vi "Main.vi"(11 "Module Admin":refnum<class "Delacor_lib_QMH_Module Admin.lvclass">) -> ()   [LabVIEW 2024, in "Coffee Prefers.lvlib"]
doc: "This template is based off of the Queued Message Handler design pattern and the Queued Message Handler project template that ships with LabVIEW.\n\nThe main difference is that the queue is private to this module and communication between modules is performed via Broadcast and Request events.\n\nRequest events are wrapped in public API methods and are handled in the Event Handling Loop (EHL) of this VI. Any module can register for Broadcast events sent by this module. The EHL generates messages based on user interface actions.\n\nThe Message Handling Loop (MHL) processes messages generated by the EHL, or by other messages. The messages are string values, so new messages can be added easily to the Message Cases case structure in the MHL. Each message cluster can also provide an optional value for Message Data, which is a variant that can be converted to whatever message-specific data is required.\n_____\nBased on DQMH Project Template 7.0.1.1316."
uses:
  Coffee Prefers.lvlib
  <vilib>/Delacor/Delacor QMH/Libraries/Module Admin_class/Delacor_lib_QMH_Module Admin.lvclass
  choose coffee--combobox.ctl
  Module Data--cluster.ctl
  <vilib>/Delacor/Delacor QMH/Libraries/Message Queue_class/Delacor_lib_QMH_Message Queue.lvclass/Delacor_lib_QMH_Message Queue.ctl
  Stop Argument--cluster.ctl
  <vilib>/Delacor/Delacor QMH/Libraries/Module Admin_class/Delacor_lib_QMH_Module Admin.lvclass/Delacor_lib_QMH_Module Admin.ctl
  user inputs--cluster.ctl
  Material broadcast -- cluster.ctl
  <vilib>/Utility/miscctls.llb/LVPointTypeDef.ctl
  <vilib>/Delacor/Delacor QMH/Libraries/Message Queue_class/Delacor_lib_QMH_Enqueue Message (Single).vi
  <vilib>/Delacor/Delacor QMH/Libraries/Module Admin_class/Delacor_lib_QMH_Get External Launch.vi
  <vilib>/Delacor/Delacor QMH/Libraries/Message Queue_class/Delacor_lib_QMH_Message Queue.lvclass
  Tank/Tank.lvlib
panel:
  in  "Milk intensity":dbl
  in  "Coffe intensity":dbl
  in  "Choose Coffe":T1
  out "error out":errorcluster
  out "Status":string
  in  "Simulate MHL Error":bool
  in  "Simulate EHL Error":bool
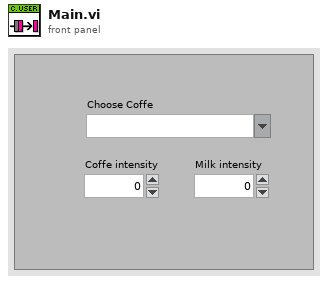
[diagram p1: front panel]
types:
  T1 = typedef "Coffee Prefers.lvlib/choose coffee--combobox.ctl" = string
  T2 = typedef "Coffee Prefers.lvlib/Request Events--cluster.ctl" = cluster{"Stop Module":refnum<user-event>, "Show Panel":refnum<user-event>, "Hide Panel":refnum<user-event>, "Get Module Execution Status":refnum<user-event>, "Show Diagram":refnum<user-event>}
  T3 = typedef "Tank.lvlib/Broadcast Events--cluster.ctl" = cluster{"Module Did Init":refnum<user-event>, "Status Updated":refnum<user-event>, "Error Reported":refnum<user-event>, "Module Did Stop":refnum<user-event>, "Update Module Execution Status":refnum<user-event>, "Tank Situation":refnum<user-event>}
  T4 = typedef "Coffee Prefers.lvlib/Module Data--cluster.ctl" = cluster{"Status":string, "Coffee":i16, "Milk":i16, "Water":i16, "milk intensity":dbl, "coffee instensity":dbl, "choose coffe":string}
  T5 = enum32{"invalid lock state", "Not Locked", "Locked (No Password)", "Password-protected"}
  T6 = typedef "Coffee Prefers.lvlib/Stop Argument--cluster.ctl" = cluster{"Origin":string, "Exit via Stop Module Req?":bool, "Wait for Module to stop?":bool}
  T7 = typedef "Coffee Prefers.lvlib/user inputs--cluster.ctl" = cluster{"choose coffe":string, "coffee instensity":dbl, "milk intensity":dbl}
  T8 = typedef "Material broadcast -- cluster.ctl" = cluster{"Coffee":i32, "Milk":i32, "Water":i32}
  T9 = typedef "LVPointTypeDef.ctl" = cluster{"Horizontal":i16, "Vertical":i16}
  T10 = enum32{"Invalid", "Standard", "Closed", "Hidden", "Minimized", "Maximized"}
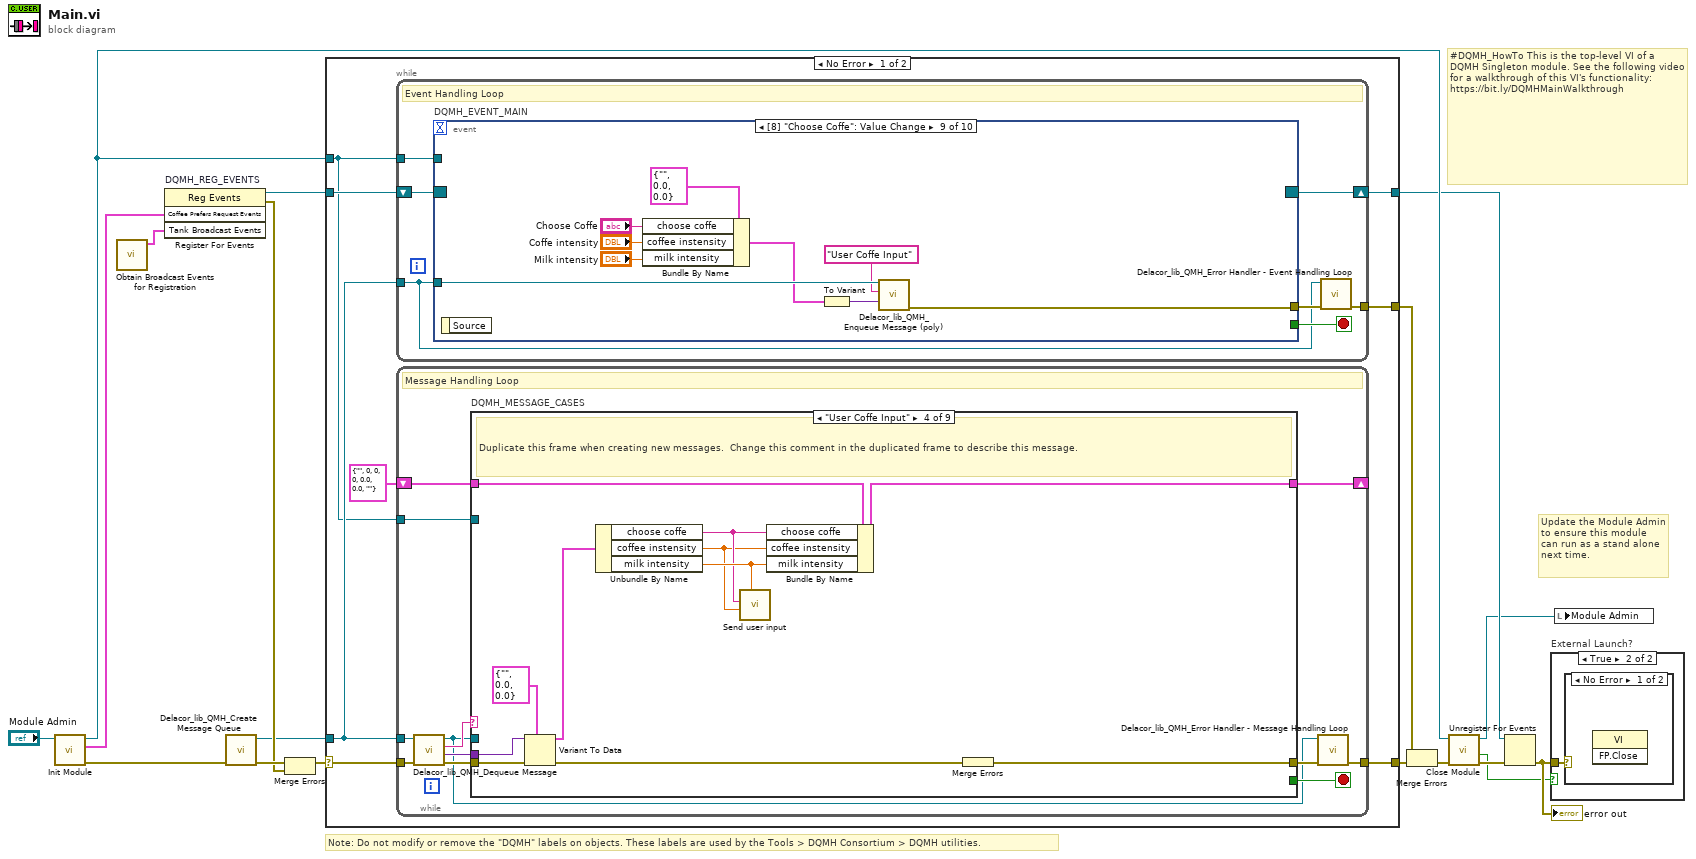
[diagram p0: block diagram]
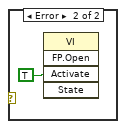
[diagram p3: hidden frame]
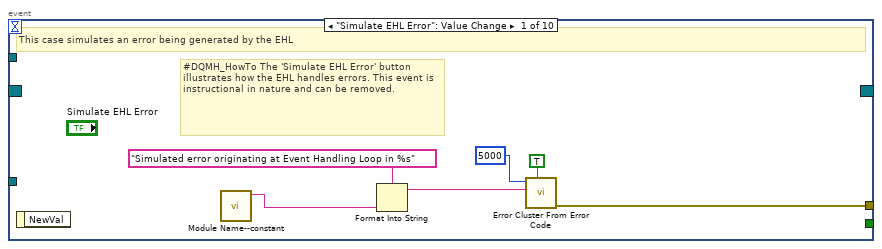
[diagram p4: hidden frame]
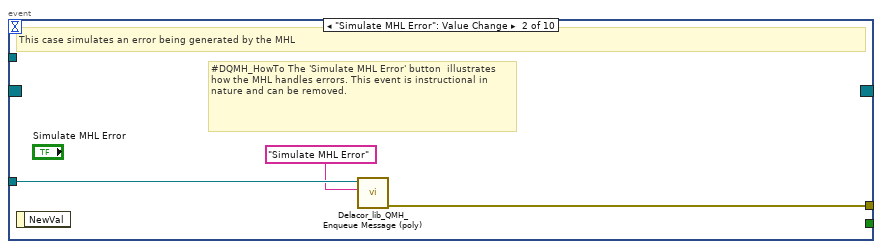
[diagram p5: hidden frame]
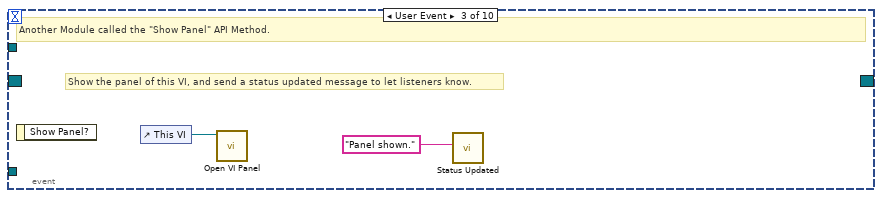
[diagram p6: hidden frame]
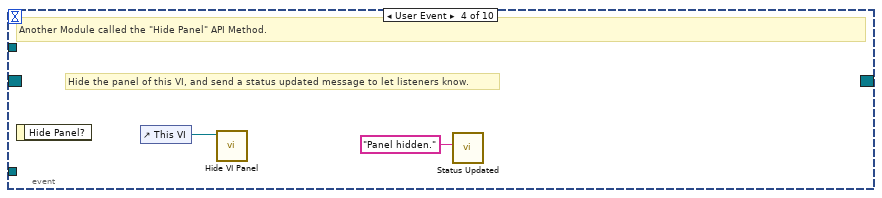
[diagram p7: hidden frame]
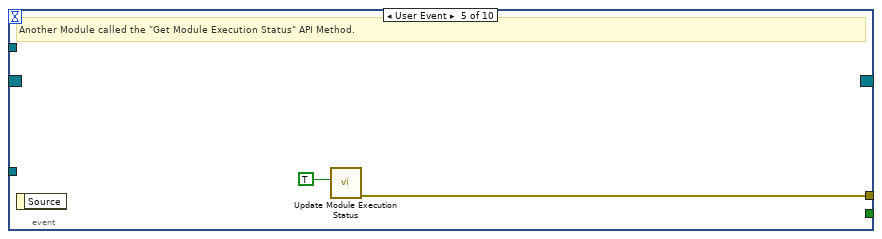
[diagram p8: hidden frame]
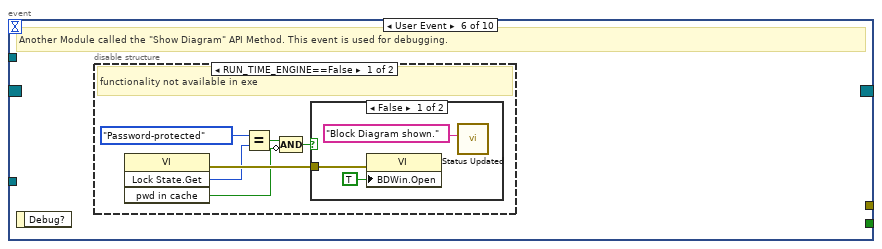
[diagram p9: hidden frame]
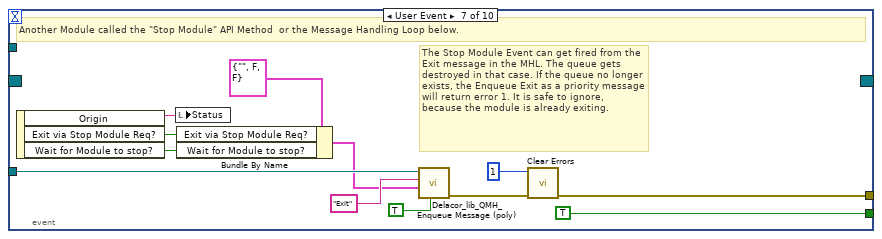
[diagram p12: hidden frame]
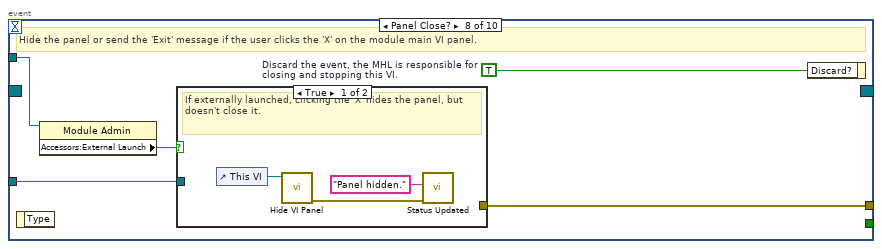
[diagram p13: hidden frame]
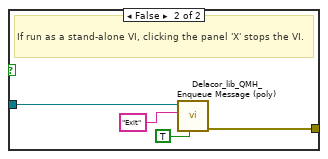
[diagram p14: hidden frame]
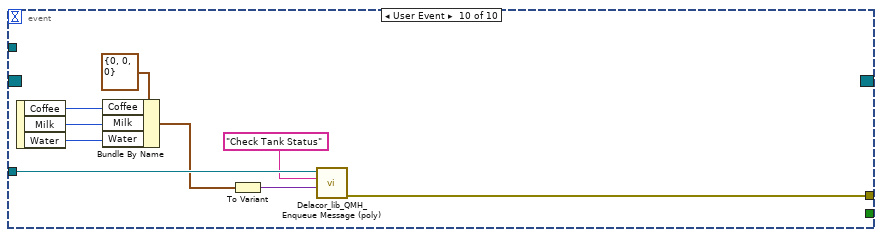
[diagram p15: hidden frame]
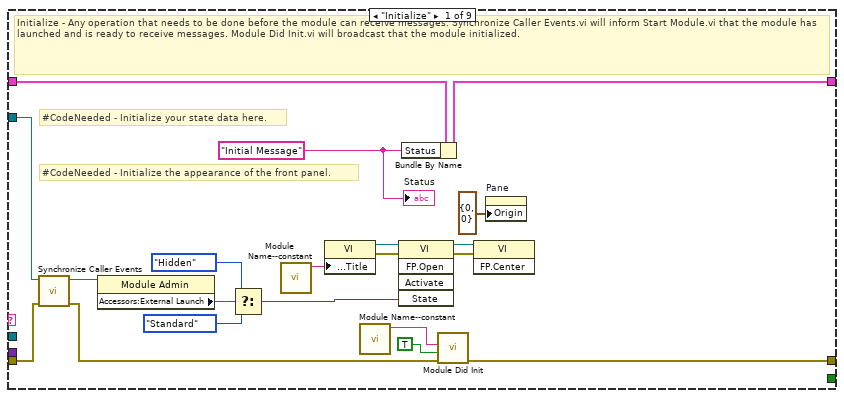
[diagram p16: hidden frame]
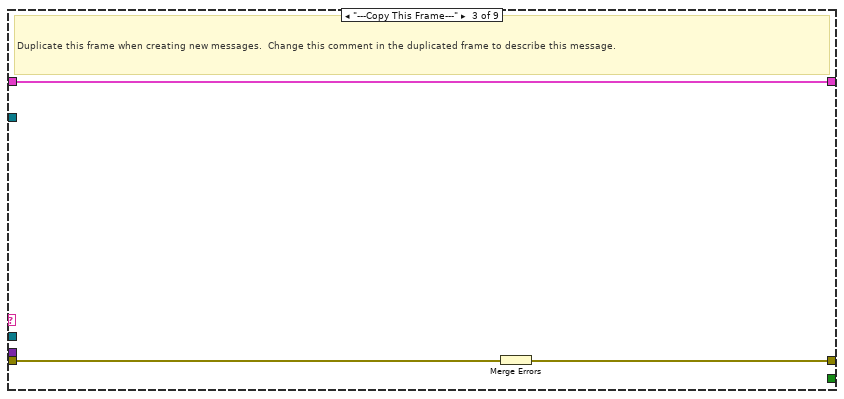
[diagram p18: hidden frame]
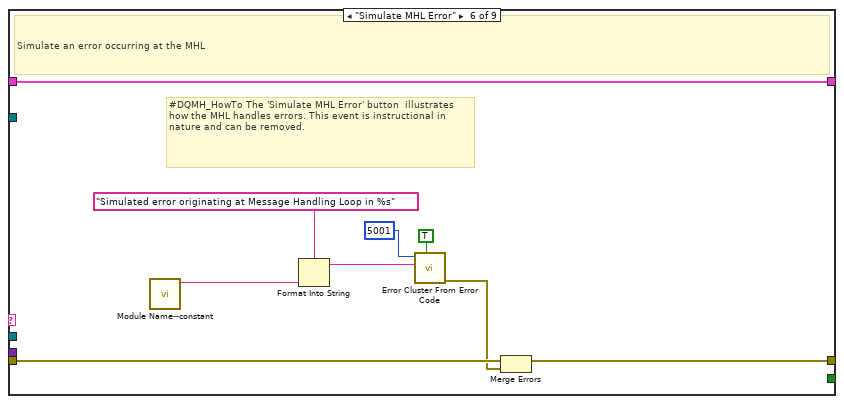
[diagram p20: hidden frame]
diagram:
  # "#DQMH_HowTo This is the top-level VI of a DQMH Singleton module. See the following video for a walkthrough of this VI's functionality: https://bit.ly/DQMHMainWalkthrough"
  # "Note: Do not modify or remove the \"DQMH\" labels on objects. These labels are used by the Tools > DQMH Consortium > DQMH utilities."
  # "Update the Module Admin to ensure this module can run as a stand alone next time."
  n1 = call "Init Module.vi"("Singleton Module Admin in"="Module Admin") -> ("error out"=w17:errorcluster, "Coffee Prefers Request Events"=w6:T2, "Singleton Module Admin out"=w9:refnum<class "Delacor_lib_QMH_Module Admin.lvclass">)  [unwired: 8 in]
  n2 = call "Obtain Broadcast Events for Registration.vi"() -> ("Tank Broadcast Events"=w1:T3)  [unwired: 9 in, 2 out]
  n3 = register-events "DQMH_REG_EVENTS"(w6, w1) -> (reference out=w7:refnum<event-registration>, error out=w10:errorcluster)  [unwired: 2 in]
  n4 = call <vilib>:"Delacor_lib_QMH_Create Message Queue.vi"("error in"=w17) -> ("error out"=w12:errorcluster, "Message Queue"=w5:refnum<class "Delacor_lib_QMH_Message Queue.lvclass">)  [unwired: 9 in]
  n5 = Merge Errors(w12, w10) -> (w11:errorcluster)
  n6 = case shown="No Error" w11 {
    selector: w11 -> [w24 w208]
    tunnel: [w26 w207] -> w18
    tunnel: [w23 w206] -> w8
    tunnel: w7 -> [w21 w206]
    tunnel: w5 -> [w20 w201]
    tunnel: [w25 _] -> w15
    tunnel: w9 -> [w19 w202]
    frame No Error {
      n7 = while {
        tunnel: w20 -> [w27]
        shift-right: [w30] -> w23
        shift-left: w21 -> [w31]
        tunnel: [w32] -> w25
        tunnel: w19 -> [w28]
        stop <- w29 stop-if-true
        # "Event Handling Loop"
        n8 = event "DQMH_EVENT_MAIN" shown="[8] \"Choose Coffe\": Value Change" {
          selector: w31 -> [_ _ _ _ _ _ _ _ _ _]
          dyn-events: [_ _ _ _ _ _ _ _ _ _] -> w30
          timeout: _ -> [_ _ _ _ _ _ _ _ _ _]
          tunnel: [_ _ _ _ _ _ TRUE ("Discard?") _ _ _] -> w29
          tunnel: w27 -> [_ w41 _ _ _ _ w65 w72 w90 w99]
          tunnel: [w39 w42 _ _ w48 _ w68 w74 w89 w98] -> w33
          tunnel: w28 -> [_ _ _ _ _ _ _ w71 _ _]
          event "Simulate EHL Error": Value Change {
            # "#DQMH_HowTo The 'Simulate EHL Error' button  illustrates how the EHL handles errors. This event is instructional in nature and can be removed."
            # "This case simulates an error being generated by the EHL"
            n9 = event-data() -> ()  [unwired: 1 in, 1 out]
            n10 = call "Module Name--constant.vi"() -> ("Module Name"=w36:string)  [unwired: 11 in]
            n11 = Format Into String(format string="Simulated error originating at Event Handling Loop in %s", w36) -> (resulting string=w37:string)  [unwired: 2 in, 1 out]
            n12 = call <vilib>:"Error Cluster From Error Code.vi"("show call chain? (False)"=TRUE, "error message (\"\")"=w37, "error code (0)"=5000) -> ("error out"=w39:errorcluster)  [unwired: 6 in]
          }
          event "Simulate MHL Error": Value Change {
            # "#DQMH_HowTo The 'Simulate MHL Error' button  illustrates how the MHL handles errors. This event is instructional in nature and can be removed."
            # "This case simulates an error being generated by the MHL"
            n13 = event-data() -> ()  [unwired: 1 in, 1 out]
            n14 = call-poly <vilib>:"Delacor_lib_QMH_Enqueue Message (poly).vi"("Message"="Simulate MHL Error", "Message Queue in"=w41) -> ("error out"=w42:errorcluster)  [unwired: 8 in, 1 out]
          }
          event User Event {
            # "Show the panel of this VI, and send a status updated message to let listeners know."
            # "Another Module called the \"Show Panel\" API Method."
            n15 = event-data() -> ()  [unwired: 1 in, 1 out]
            n16 = control-ref of="This VI"() -> (w44:refnum<vi>)
            n17 = call "Open VI Panel.vi"("VI"=w44) -> ()  [unwired: 10 in, 1 out]
            n18 = call "Status Updated.vi"("Status"="Panel shown." ("format string")) -> ()  [unwired: 10 in, 1 out]
          }
          event User Event {
            # "Hide the panel of this VI, and send a status updated message to let listeners know."
            # "Another Module called the \"Hide Panel\" API Method."
            n19 = event-data() -> ()  [unwired: 1 in, 1 out]
            n20 = control-ref of="This VI"() -> (w46:refnum<vi>)
            n21 = call "Hide VI Panel.vi"("VI"=w46) -> ()  [unwired: 10 in, 1 out]
            n22 = call "Status Updated.vi"("Status"="Panel hidden." ("format string")) -> ()  [unwired: 10 in, 1 out]
          }
          event User Event {
            # "Another Module called the \"Get Module Execution Status\" API Method."
            n23 = event-data() -> ()  [unwired: 1 in, 1 out]
            n24 = call "Update Module Execution Status.vi"("Running?"=TRUE) -> ("error out"=w48:errorcluster)  [unwired: 10 in]
          }
          event User Event {
            # "Another Module called the \"Show Diagram\" API Method. This event is used for debugging."
            n25 = event-data() -> ()  [unwired: 1 in, 1 out]
            n26 = disable-structure shown="RUN_TIME_ENGINE==False" {
              frame condition #0 (active) {
                # "functionality not available in exe"
                n27 = invoke on="Invoke Node" class="VI" method="Lock State.Get"() -> (error out=w54:errorcluster, "Get Lock State"=w53:T5, "pwd in cache"=w50:bool)  [unwired: 4 in, 1 out]
                n28 = Equal?(x=T5."Password-protected", y=w53) -> (x = y?=w51:bool)
                n29 = Compound Arithmetic op=AND(w51, invert w50) -> (w49:bool)
                n30 = case shown="False" w49 {
                  tunnel: w54 -> [w57 _]
                  frame False {
                    n31 = property on="Property Node" class="VI"(error in=w57, "BDWin.Open"=TRUE ("Block Diagram Window:Open")) -> ()  [unwired: 1 in, 2 out]
                    n32 = call "Status Updated.vi"("Status"="Block Diagram shown." ("format string")) -> ()  [unwired: 10 in, 1 out]
                  }
                  frame True {
                    # "Password-protected VI, and the password is not in the cache. Do not show the diagram."
                  }
                }
              }
              frame condition #1 {
              }
            }
          }
          event User Event {
            # "The Stop Module Event can get fired from the Exit message in the MHL. The queue gets destroyed in that case. If the queue no longer exists, the Enqueue Exit as a priority message will return error 1. It is safe to ignore, because the module is already exiting."
            # "Another Module called the \"Stop Module\" API Method  or the Message Handling Loop below."
            n33 = event-data() -> ("Origin"=w64:string, "Exit via Stop Module Req?"=w60:bool, "Wait for Module to stop?"=w59:bool)  [unwired: 1 in]
            n34 = local write "Status"(w64) -> ()
            n35 = Bundle By Name(cluster=T6 {"Origin"="", "Exit via Stop Module Req?"=FALSE, "Wait for Module to stop?"=FALSE} ("Stop Argument"), "Exit via Stop Module Req?"=w60, "Wait for Module to stop?"=w59) -> (w58:T6)
            n36 = call-poly <vilib>:"Delacor_lib_QMH_Enqueue Message (poly).vi"("Priority Message? (F)"=TRUE, "Message Data"=w58, "Message"="Exit", "Message Queue in"=w65) -> ("error out"=w69:errorcluster)  [unwired: 6 in, 1 out]
            n37 = call <vilib>:"Clear Errors.vi"("error in (no error)"=w69, "specific error code to clear (0: all)"=1) -> ("error out"=w68:errorcluster)  [unwired: 4 in, 1 out]
          }
          event Panel Close? {
            w73 = TRUE  # Discard the event, the MHL is responsible for closing and stopping this VI.
            # "Hide the panel or send the 'Exit' message if the user clicks the 'X' on the module main VI panel."
            n38 = event-data() -> ()  [unwired: 1 in, 1 out]
            n39 = property on="Property Node" class="Module Admin"(reference=w71) -> ("Accessors:External Launch"=w70:bool)  [unwired: 1 in, 2 out]
            n40 = case shown="True" w70 {
              tunnel: w72 -> [_ w80]
              tunnel: [_ w81] -> w74
              frame True {
                # "If externally launched, clicking the 'X' hides the panel, but doesn't close it."
                n41 = control-ref of="This VI"() -> (w77:refnum<vi>)
                n42 = call "Hide VI Panel.vi"("VI"=w77) -> ("error out"=w75:errorcluster)  [unwired: 10 in]
                n43 = call "Status Updated.vi"("error in"=w75, "Status"="Panel hidden." ("format string")) -> ()  [unwired: 9 in, 1 out]
              }
              frame False {
                # "If run as a stand-alone VI, clicking the panel 'X' stops the VI."
                n44 = call-poly <vilib>:"Delacor_lib_QMH_Enqueue Message (poly).vi"("Priority Message? (F)"=TRUE, "Message"="Exit", "Message Queue in"=w80) -> ("error out"=w81:errorcluster)  [unwired: 7 in, 1 out]
              }
            }
            n45 = event-data ("Event Filter Node")("Discard?"=w73) -> ()  [unwired: 1 in, 1 out]
          }
          event Value Change {
            n46 = event-data() -> ()  [unwired: 1 in, 1 out]
            n47 = Bundle By Name(cluster=T7 {"choose coffe"="", "coffee instensity"=0.0, "milk intensity"=0.0}, "choose coffe"="Choose Coffe", "coffee instensity"="Coffe intensity", "milk intensity"="Milk intensity") -> (w82:T7)
            n48 = To Variant(anything=w82) -> (Variant=w83:variant)
            n49 = call-poly <vilib>:"Delacor_lib_QMH_Enqueue Message (poly).vi"("Message Data"=w83, "Message"="User Coffe Input", "Message Queue in"=w90) -> ("error out"=w89:errorcluster)  [unwired: 7 in, 1 out]
          }
          event User Event {
            n50 = event-data() -> ("Coffee"=w96:i16, "Milk"=w95:i16, "Water"=w94:i16)  [unwired: 1 in]
            n51 = Bundle By Name(cluster=T8 {"Coffee"=0, "Milk"=0, "Water"=0}, "Coffee"=w96, "Milk"=w95, "Water"=w94) -> (w92:T8)
            n52 = To Variant(anything=w92) -> (Variant=w93:variant)
            n53 = call-poly <vilib>:"Delacor_lib_QMH_Enqueue Message (poly).vi"("Message Data"=w93, "Message"="Check Tank Status", "Message Queue in"=w99) -> ("error out"=w98:errorcluster)  [unwired: 7 in, 1 out]
          }
        }
        n54 = call-dynamic "Delacor_lib_QMH_Error Handler - Event Handling Loop.vi"("error in"=w33, "Message Queue in"=w27) -> ("dup error in"=w32:errorcluster)  [unwired: 8 in, 1 out]
      }
      n55 = while {
        tunnel: w20 -> [w100]
        shift-right: [w108] -> _
        shift-left: T4 {"Status"="", "Coffee"=0, "Milk"=0, "Water"=0, "milk intensity"=0.0, "coffee instensity"=0.0, "choose coffe"=""} ("Data Cluster") -> [w109]
        tunnel: w24 -> [w111]
        tunnel: [w103] -> w26
        tunnel: w19 -> [w104]
        stop <- w107 stop-if-true
        # "Message Handling Loop"
        n56 = call-dynamic "Delacor_lib_QMH_Dequeue Message.vi"("error in"=w111, "Message Queue in"=w100) -> ("error out"=w110:errorcluster, "Message Data"=w105:variant, "Message"=w106:string, "Message Queue out"=w101:refnum<class "Delacor_lib_QMH_Message Queue.lvclass">)  [unwired: 6 in]
        n57 = case "DQMH_MESSAGE_CASES" shown="\"User Coffe Input\"" w106 {
          selector: w106 -> [_ _ _ _ _ _ _ _ w196]
          tunnel: w101 -> [_ _ _ _ _ _ w162 w184 _]
          tunnel: w110 -> [w129 w133 w136 w147 w149 w158 w169 w190 w199]
          tunnel: [w127 w133 w135 w146 w149 w157 w165 w185 w200] -> w102
          tunnel: w109 -> [w118 w132 w134 w141 w148 w155 w164 w183 w197]
          tunnel: [w117 w132 w134 w140 w148 w155 w164 w183 w197] -> w108
          tunnel: [_ _ _ _ _ _ _ w182 _] -> w107
          tunnel: w105 -> [_ _ _ w143 _ _ w163 w181 _]
          tunnel: w104 -> [w119 _ _ _ _ _ w161 w176 _]
          frame "Initialize" {
            w113 = "Initial Message" ("Initial Message")
            # "#CodeNeeded - Initialize the appearance of the front panel."
            # "#CodeNeeded - Initialize your state data here."
            # "Initialize - Any operation that needs to be done before the module can receive messages. Synchronize Caller Events.vi will inform Start Module.vi that the module has launched and is ready to receive messages. Module Did Init.vi will broadcast that the module initialized."
            n58 = call "Synchronize Caller Events.vi"("error in"=w129, "Singleton Module Admin in"=w119) -> ("error out"=w128:errorcluster, "Singleton Module Admin out"=w114:refnum<class "Delacor_lib_QMH_Module Admin.lvclass">)  [unwired: 8 in]
            n59 = property on="Property Node" class="Module Admin"(reference=w114) -> ("Accessors:External Launch"=w123:bool)  [unwired: 1 in, 2 out]
            n60 = Select(t=T10."Hidden" ("State"), s=w123, f=T10."Standard" ("State")) -> (s? t:f=w120:T10)
            n61 = call "Module Name--constant.vi"() -> ("Module Name"=w126:string)  [unwired: 11 in]
            n62 = property on="Property Node" class="VI"("Front Panel.Title"=w126) -> (reference out=w125:refnum<vi>, error out=w131:errorcluster)  [unwired: 2 in]
            n63 = call "Module Name--constant.vi"() -> ("Module Name"=w115:string)  [unwired: 11 in]
            n64 = invoke on="Invoke Node" class="VI" method="FP.Open"(reference=w125, error in=w131, "State"=w120) -> (reference out=w124:refnum<vi>, error out=w130:errorcluster)  [unwired: 2 in, 3 out]
            n65 = Bundle By Name(cluster=w118, "Status"=w113) -> (w117:T4)
            n66 = call "Module Did Init.vi"("error in"=w128, "Initialized?"=TRUE, "Origin"=w115) -> ("error out"=w127:errorcluster)  [unwired: 8 in]
            n67 = invoke on="Invoke Node" class="VI" method="FP.Center"(reference=w124, error in=w130) -> ()  [unwired: 1 in, 3 out]
            n68 = property on="Pane" class="Pane"("Origin"=T9 {"Horizontal"=0, "Vertical"=0}) -> ()  [unwired: 2 in, 2 out]
            "Status" <- w113
          }
          frame "---Module Specific---" {
            # "Separator -- The following cases handle messages specific to this Module."
          }
          frame "---Copy This Frame---" {
            # "Duplicate this frame when creating new messages.  Change this comment in the duplicated frame to describe this message."
            n69 = Merge Errors(w136) -> (w135:errorcluster)
          }
          frame "User Coffe Input" {
            # "Duplicate this frame when creating new messages.  Change this comment in the duplicated frame to describe this message."
            n70 = Variant To Data(error in=w147, type=T7 {"choose coffe"="", "coffee instensity"=0.0, "milk intensity"=0.0}, Variant=w143) -> (data=w142:T7, error out=w145:errorcluster)
            n71 = Unbundle By Name(w142) -> ("choose coffe"=w138:string, "coffee instensity"=w137:dbl, "milk intensity"=w139:dbl)
            n72 = call "Send user input.vi"("Milk intensity"=w139, "Coffe intensity"=w137, "Choose Coffee"=w138) -> ()  [unwired: 8 in, 1 out]
            n73 = Bundle By Name(cluster=w141, "choose coffe"=w138, "coffee instensity"=w137, "milk intensity"=w139) -> (w140:T4)
            n74 = Merge Errors(w145) -> (w146:errorcluster)
          }
          frame "---Exit and Error Handling---" {
            # "Separator - The following cases handle errors and exit messages."
          }
          frame "Simulate MHL Error" {
            # "#DQMH_HowTo The 'Simulate MHL Error' button  illustrates how the MHL handles errors. This event is instructional in nature and can be removed."
            # "Simulate an error occurring at the MHL"
            n75 = call "Module Name--constant.vi"() -> ("Module Name"=w151:string)  [unwired: 11 in]
            n76 = Format Into String(format string="Simulated error originating at Message Handling Loop in %s", w151) -> (resulting string=w152:string)  [unwired: 2 in, 1 out]
            n77 = call <vilib>:"Error Cluster From Error Code.vi"("show call chain? (False)"=TRUE, "error message (\"\")"=w152, "error code (0)"=5001) -> ("error out"=w156:errorcluster)  [unwired: 6 in]
            n78 = Merge Errors(w158, w156) -> (w157:errorcluster)
          }
          frame "Error" {
            # "#CodeRecommended - If the module is running in standalone mode (External Launch = FALSE), this code will pop up an error dialog and call the 'Exit' message if an error occurs. Add more fine-grained error management here."
            # "Error - Check the error message data and respond accordingly. This message is sent by the \"Error Handler\" VIs at the end of each loop in this application."
            n79 = property on="Property Node" class="Module Admin"(reference=w161) -> ("Accessors:External Launch"=w160:bool)  [unwired: 1 in, 2 out]
            n80 = Variant To Data(error in=w169, type=errorcluster {"status"=FALSE, "code"=0, "source"=""} ("error constant"), Variant=w163) -> (data=w159:errorcluster, error out=w167:errorcluster)
            n81 = local write "error out"(w159) -> ()
            n82 = call "Error Reported.vi"("Error"=w159) -> ()  [unwired: 10 in, 1 out]
            n83 = case shown="False" w160 {
              tunnel: [w174 _] -> w166
              tunnel: w162 -> [w172 _]
              tunnel: w159 -> [w173 _]
              frame False {
                n84 = disable-structure shown="Default" {
                  disable-tunnel: w173 -> [w175 _]
                  frame condition #0 (active) {
                    # "If the module is running standalone, then pop up an error dialog and call the \"Exit\" message."
                    n85 = call <vilib>:"Simple Error Handler.vi"("error in (no error)"=w175) -> ()  [unwired: 4 in, 5 out]
                  }
                  frame condition #1 {
                    # "To prevent the Simple Error Handler VI from being loaded (e.g. when deploying to a Real-Time target), add the Conditional Disable Symbol \"DQMH_Disable_SEH\" to your project and set it to TRUE."
                  }
                }
                n86 = call-poly <vilib>:"Delacor_lib_QMH_Enqueue Message (poly).vi"("Priority Message? (F)"=TRUE, "Message"="Exit", "Message Queue in"=w172) -> ("error out"=w174:errorcluster)  [unwired: 7 in, 1 out]
              }
              frame True {
                # "If the module was launched externally, calling the Error Reported broadcast VI is the only action performed by the \"Error\" message. The module's caller can then process the error appropriately."
              }
            }
            n87 = Merge Errors(w167, w166) -> (w165:errorcluster)
          }
          frame "Exit" {
            w180 = 91  # 91: not all Exit messages will have an argument
            w182 = TRUE  # Stop the VI
            # "Release the message queue reference"
            # "#CodeNeeded - Add any required cleanup code here."
            # "Exit - Exit the application."
            n88 = Variant To Data(error in=w190, type=T6 {"Origin"="", "Exit via Stop Module Req?"=FALSE, "Wait for Module to stop?"=FALSE} ("Stop Argument"), Variant=w181) -> (data=w178:T6, error out=w187:errorcluster)
            n89 = call <vilib>:"Clear Errors.vi"("error in (no error)"=w187, "specific error code to clear (0: all)"=w180) -> ("error out"=w189:errorcluster)  [unwired: 4 in, 1 out]
            n90 = control-ref of="This VI"() -> (w177:refnum<vi>)
            n91 = call-dynamic "Delacor_lib_QMH_Release Message Queue.vi"("error in"=w189, "Message Queue"=w184) -> ("error out"=w188:errorcluster)  [unwired: 9 in]
            n92 = call "Handle Exit.vi"("Stop Argument"=w178, "Admin in"=w176, "VI reference"=w177) -> ("error out"=w186:errorcluster)  [unwired: 7 in, 1 out]
            n93 = Merge Errors(w188, w186) -> (w185:errorcluster)
            n94 = call "Error Reported.vi"("Error"=w185) -> ()  [unwired: 10 in, 1 out]
          }
          frame Default {
            # "'Default' case only runs if there is a message that isn't defined in any of the other cases.  Output a programming error."
            n95 = call "Module Name--constant.vi"() -> ("Module Name"=w195:string)  [unwired: 11 in]
            n96 = Format Into String(format string="The invalid message string \"%s\" was received in the Message Handling Loop for module \"%s\".", w196, w195) -> (resulting string=w191:string)  [unwired: 2 in, 1 out]
            n97 = call <vilib>:"Error Cluster From Error Code.vi"("show call chain? (False)"=TRUE, "error message (\"\")"=w191, "error code (0)"=1) -> ("error out"=w198:errorcluster)  [unwired: 6 in]
            n98 = Merge Errors(w199, w198) -> (w200:errorcluster)
          }
        }
        n99 = call-dynamic "Delacor_lib_QMH_Error Handler - Message Handling Loop.vi"("error in"=w102, "Message Queue in"=w101) -> ("dup error in"=w103:errorcluster)  [unwired: 8 in, 1 out]
      }
    }
    frame Error {
      # "Synchronize Caller Events.vi will inform Start Module.vi that the module has launched and will let the code calling Start Module.vi register for broadcasts and would permit the caller receive the broadcast that an error occurred at launch time."
      n100 = call-dynamic "Delacor_lib_QMH_Release Message Queue.vi"("error in"=w208, "Message Queue"=w201) -> ("error out"=w207:errorcluster)  [unwired: 9 in]
      n101 = call "Synchronize Caller Events.vi"("Singleton Module Admin in"=w202) -> ("error out"=w209:errorcluster)  [unwired: 9 in, 1 out]
      n102 = call "Module Name--constant.vi"() -> ("Module Name"=w205:string)  [unwired: 11 in]
      n103 = Format Into String(format string="An error occurred during initialization. %s is no longer running.", w205) -> (resulting string=w203:string)  [unwired: 2 in, 1 out]
      n104 = Merge Errors(w207, w209) -> (w210:errorcluster)
      n105 = call "Error Reported.vi"("Additional Information"=w203, "Error"=w210) -> ()  [unwired: 9 in, 1 out]
    }
  }
  n106 = Merge Errors(w15, w18) -> (w14:errorcluster)
  n107 = call "Close Module.vi"("error in"=w14, "Module Admin in"=w9) -> ("error out"=w16:errorcluster, "External Launch"=w2:bool, "Module Admin out"=w3:refnum<class "Delacor_lib_QMH_Module Admin.lvclass">)  [unwired: 7 in]
  n108 = Unregister For Events(event registration refnum=w8, error in=w16) -> (error out=w13:errorcluster)
  "error out" <- w13
  n109 = case "External Launch?" shown="True" w2 {
    tunnel: w13 -> [_ w211]
    frame False {
    }
    frame True {
      n110 = case shown="No Error" w211 {
        frame No Error {
          n111 = invoke on="Invoke Node" class="VI" method="FP.Close"() -> ()  [unwired: 3 in, 3 out]
        }
        frame Error {
          n112 = invoke on="Invoke Node" class="VI" method="FP.Open"("Activate"=TRUE ("Activate?")) -> ()  [unwired: 4 in, 5 out]
        }
      }
    }
  }
  n113 = local write "Module Admin"(w3) -> ()
